vi "Log Data to File.vi"(8 "error in (no error)":errorcluster, 10 "Data to log":waveform(dbl)[](array[waveform]), 11 "TDMS File Reference":refnum<k34>) -> (0 "error out":errorcluster)   [LabVIEW 2020, in "FileLogging.lvlib"]
doc: "This VI uses the TDMS Write function to write data to a TDMS file.\n_____\nBased on Delacor QMH Project Template 5.0.0.82."
uses:
  FileLogging.lvlib
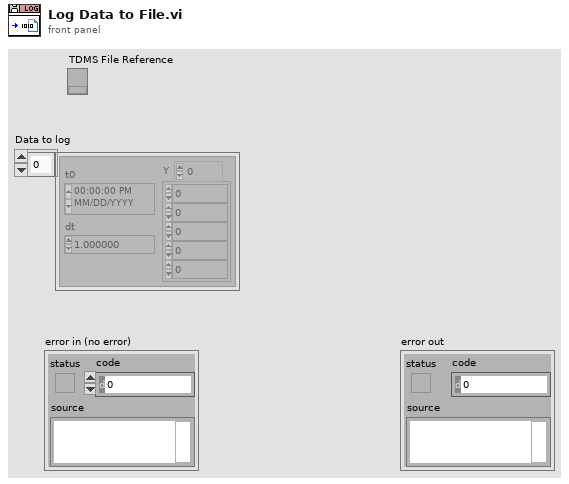
[diagram p1: front panel]
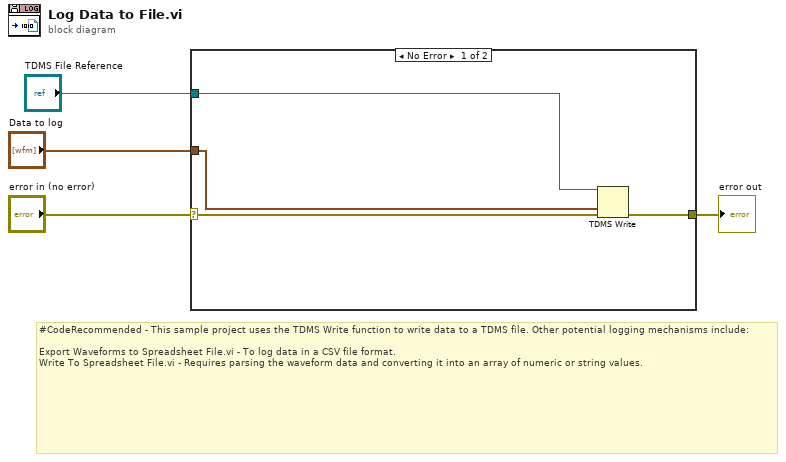
[diagram p0: block diagram]
diagram:
  # "#CodeRecommended - This sample project uses the TDMS Write function to write data to a TDMS file. Other potential logging mechanisms include:\n\nExport Waveforms to Spreadsheet File.vi - To log data in a CSV file format.\nWrite To Spreadsheet File.vi - Requires parsing the waveform data and converting it into an array of numeric or string values."
  n1 = case shown="No Error" "error in (no error)" {
    selector: "error in (no error)" -> [w7 w9]
    tunnel: "Data to log" -> [w6 _]
    tunnel: [w8 w9] -> w3
    tunnel: "TDMS File Reference" -> [w5 _]
    frame No Error {
      n2 = TDMS Write(0:w5, 9:w6, 11:w7) -> (15:w8:errorcluster)  [unwired: 3 in, 3 out]
    }
    frame Error {
    }
  }
  "error out" <- w3
